vi "Check Fan Temperature.vi"(8 "error in":errorcluster, 11 "DeepU Test Stand in":refnum<class "DeepU Test Stand.lvclass">) -> (0 "error out":errorcluster, 3 "DeepU Test Stand out":refnum<class "DeepU Test Stand.lvclass">)   [LabVIEW 2019, in "Test Stands.lvlib" / "DeepU Test Stand.lvclass"]
uses:
  DeepU Test Stand.lvclass
  Results/Results Method.ctl
  Results/DeepU Results/DeepU Results.lvclass
  DeepU Test Stand.lvclass/DeepU Test Stand.ctl
  Results/DeepU Results/DeepU Results.lvclass/DeepU Results.ctl
  <vilib>/DAQmx/read.llb/DAQmx Read (Analog DBL 1Chan 1Samp).vi
  <vilib>/DAQmx/miscellaneous.llb/DAQmx Fill In Error Info.vi
  Results/Results.lvlib
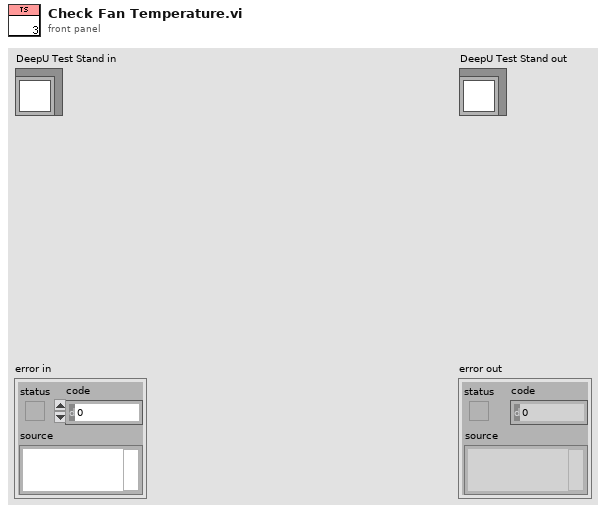
[diagram p1: front panel]
types:
  T1 = typedef "Results.lvlib/Results Method.ctl" = enum16{"Get", "Set"}
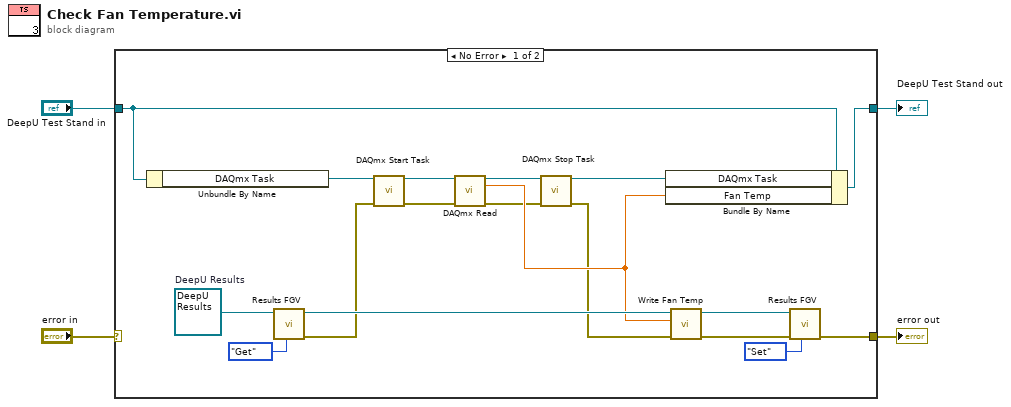
[diagram p0: block diagram]
diagram:
  n1 = case shown="No Error" "error in" {
    selector: "error in" -> [_ w24]
    tunnel: [w13 w24] -> w3
    tunnel: [w21 w23] -> w1
    tunnel: "DeepU Test Stand in" -> [w22 w23]
    frame No Error {
      w20 = refnum<class "DeepU Results.lvclass"> refnum  # DeepU Results
      n2 = Unbundle By Name(w22) -> ("DAQmx Task"=w12:refnum<k21>)
      n3 = call-dynamic "Results FGV.vi"("Method"=Results_Method."Get", "DeepU Results in"=w20) -> ("error out"=w10:errorcluster, "DeepU Results out"=w17:refnum<class "DeepU Results.lvclass">)  [unwired: 8 in]
      n4 = call <vilib>:"DAQmx Start Task.vi"("task/channels in"=w12, "error in"=w10) -> ("task out"=w11:refnum<k21>, "error out"=w9:errorcluster)  [unwired: 12 in]
      n5 = call-poly <vilib>:"DAQmx Read.vi"("task/channels in"=w11, "error in"=w9) -> ("task out"=w8:refnum<k21>, "data"=w15:dbl, "error out"=w6:errorcluster)  [unwired: 11 in]
      n6 = call <vilib>:"DAQmx Stop Task.vi"("task/channels in"=w8, "error in"=w6) -> ("task out"=w7:refnum<k21>, "error out"=w5:errorcluster)  [unwired: 12 in]
      n7 = Bundle By Name(cluster=w22, "DAQmx Task"=w7, "Fan Temp"=w15) -> (w21:refnum<class "DeepU Test Stand.lvclass">)
      n8 = call "Write Fan Temp.vi"("error in (no error)"=w5, "Fan Temp"=w15, "DeepU Results in"=w17) -> ("error out"=w14:errorcluster, "DeepU Results out"=w16:refnum<class "DeepU Results.lvclass">)  [unwired: 7 in]
      n9 = call-dynamic "Results FGV.vi"("Method"=Results_Method."Set", "error in"=w14, "DeepU Results in"=w16) -> ("error out"=w13:errorcluster)  [unwired: 7 in, 1 out]
    }
    frame Error {
    }
  }
  "error out" <- w3
  "DeepU Test Stand out" <- w1
